vi "Memory.Pointer.Parameter Check.Subset.Power of 2.vi"(5 "power of 2":i16, 7 "source vi name":string, 8 "error in (no error)":errorcluster, 9 "offset (0)":u64 format="%08x bytes", 10 "count":u64 format="%08x bytes", 11 "Pointer in":refnum<class "Memory.Pointer.lvclass">) -> (0 "error out":errorcluster, 1 "offset out":u64 format="%08x bytes", 2 "count":u64 format="%08x bytes", 3 "Pointer out":refnum<class "Memory.Pointer.lvclass">)   [LabVIEW 2016, in "Memory.lvlib" / "Memory.Pointer.lvclass"]
uses:
  Memory.Pointer.lvclass
  Memory.Pointer.lvclass/Memory.Pointer.ctl
  Memory.Pointer.Errors.Out of Bounds.vi
  Submodules/SEH/Source/VIs/Static Error Handling.Source Buffer.Write.String.vi
  Memory.Pointer.Errors.Write Pointer Size.vi
  Memory.Pointer.Errors.Create Error.vi
  Submodules/SEH/Source/VIs/Static Error Handling.Source Buffer.Write.Numeric.Scalar.Base10.vi
  Submodules/SEH/Source/VIs/Static Error Handling.Source Buffer.Write.Numeric.Scalar.Base10 (U64).vi
  Submodules/SEH/Source/VIs/Static Error Handling.Error Cluster Constant.vi
  Submodules/SEH/Source/VIs/Static Error Handling.Error Cluster Constant (256B).vi
  Submodules/SEH/Source/VIs/Static Error Handling.Parameters.Status.Set.vi
  Submodules/SEH/Source/VIs/Static Error Handling.Parameters.Code.Set.vi
  Submodules/SEH/Source/VIs/Static Error Handling.Parameters.VI Source.Set.vi
  Constants/Memory.Constants.vi
  Constants/Memory.Constants.Library Name.vi
  Memory.Pointer.Errors.Get Info.vi
  Memory.lvlib
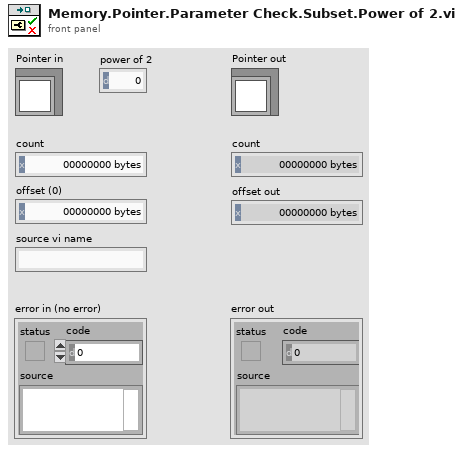
[diagram p1: front panel]
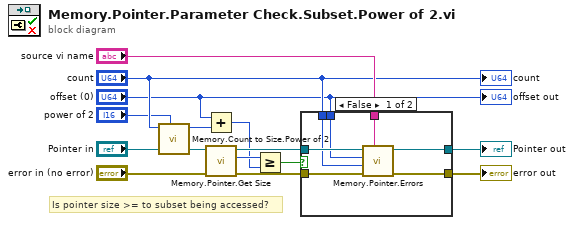
[diagram p0: block diagram]
diagram:
  # "Is pointer size >= to subset being accessed?"
  n1 = call "Memory.Count to Size.Power of 2.vi"("power of 2"="power of 2", "count"="count") -> ("size"=w3:u64)  [unwired: 9 in]
  n2 = Add(x="offset (0)", y=w3) -> (x+y=w1:u64)
  n3 = call "Memory.Pointer.Get Size.vi"("error in (no error)"="error in (no error)", "Pointer in"="Pointer in") -> ("error out"=w9:errorcluster, "size"=w12:u64, "Pointer out"=w7:refnum<class "Memory.Pointer.lvclass">)  [unwired: 7 in]
  n4 = Greater Or Equal?(x=w12, y=w1) -> (x >= y?=w8:bool)
  n5 = case shown="False" w8 {
    tunnel: w7 -> [w21 w22]
    tunnel: w9 -> [w19 w23]
    tunnel: [w18 w23] -> w14
    tunnel: [w20 w22] -> w13
    tunnel: "offset (0)" -> [w17 _]
    tunnel: "count" -> [w16 _]
    tunnel: "source vi name" -> [w15 _]
    frame False {
      n6 = call-poly "Memory.Pointer.Errors.vi"("source vi name"=w15, "error in (no error)"=w19, "length"=w16, "offset"=w17, "pointer in"=w21) -> ("error out"=w18:errorcluster, "pointer out"=w20:refnum<class "Memory.Pointer.lvclass">)  [unwired: 5 in]
    }
    frame True {
    }
  }
  "error out" <- w14
  "Pointer out" <- w13
  "offset out" <- "offset (0)"
  "count" <- "count"
